vi "CreateWO-CreateFolderOnNetwork.vi"(8 "error in (no error)":errorcluster, 9 "Sales Order":string="1234", 10 "Work Order":string="1234", 11 "NI_report in":refnum<class "NI_report.lvclass">) -> (0 "error out":errorcluster, 1 "Work Order":string, 2 "Path for Saving the file":path, 3 "NI_report out":refnum<class "NI_report.lvclass">, 5 "Path for Outlook":path)   [LabVIEW 2013, in "ERP-CreateWorkOrder.lvclass"]
uses:
  ERP-CreateWorkOrder.lvclass
  <vilib>/Utility/NIReport.llb/NI_report.lvclass
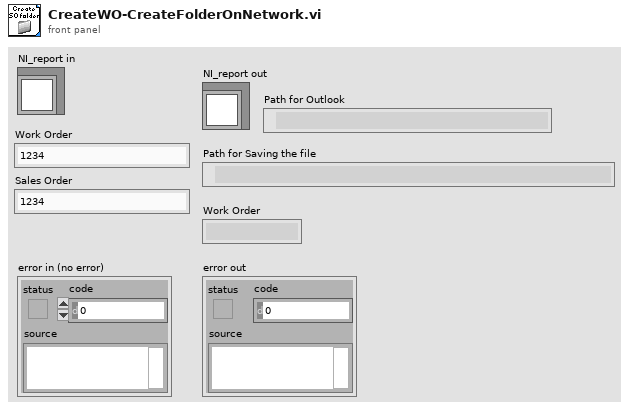
[diagram p1: front panel]
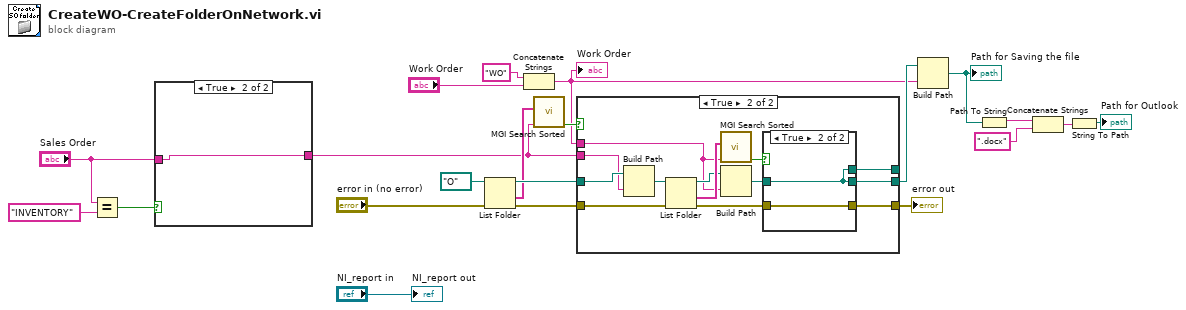
[diagram p0: block diagram]
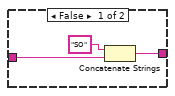
[diagram p2: hidden frame]
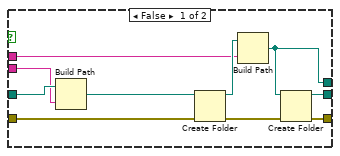
[diagram p3: hidden frame]
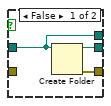
[diagram p4: hidden frame]
diagram:
  n1 = Equal?(x="Sales Order", y="INVENTORY") -> (x = y?=w6:bool)
  n2 = case shown="True" w6 {
    tunnel: "Sales Order" -> [w23 w25]
    tunnel: [w22 w25] -> w12
    frame False {
      n3 = Concatenate Strings("SO" ("string"), w23) -> (w22:string)
    }
    frame True {
    }
  }
  n4 = List Folder(path=path "O:/" ("base path"), error in="error in (no error)") -> (path out=w18:path, folder names=w14:string[], error out=w19:errorcluster)  [unwired: 2 in, 1 out]
  n5 = Concatenate Strings("WO" ("string"), "Work Order") -> (w9:string)
  "Work Order" <- w9
  n6 = call <userlib>:"MGI Search Sorted.vi"("Search String"=w12, "Sorted Strings"=w14) -> ("Found"=w13:bool)  [unwired: 6 in, 3 out]
  n7 = case shown="True" w13 {
    tunnel: w19 -> [w32 w44]
    tunnel: w18 -> [w34 w46]
    tunnel: [w27 w48] -> w17
    tunnel: [w28 w47] -> w16
    tunnel: w9 -> [w29 w38]
    tunnel: w12 -> [w33 w45]
    tunnel: [w26 w36] -> _
    frame False {
      n8 = Build Path(base path=w34, name or relative path=w33) -> (appended path=w35:path)
      n9 = Create Folder(path (use dialog)=w35, error in=w32) -> (created path=w30:path, error out=w31:errorcluster)  [unwired: 1 in, 1 out]
      n10 = Build Path(base path=w30, name or relative path=w29) -> (appended path=w26:path)
      n11 = Create Folder(path (use dialog)=w26, error in=w31) -> (created path=w28:path, error out=w27:errorcluster)  [unwired: 1 in, 1 out]
    }
    frame True {
      n12 = Build Path(base path=w46, name or relative path=w45) -> (appended path=w40:path)
      n13 = List Folder(path=w40, error in=w44) -> (path out=w39:path, folder names=w43:string[], error out=w41:errorcluster)  [unwired: 2 in, 1 out]
      n14 = call <userlib>:"MGI Search Sorted.vi"("Search String"=w38, "Sorted Strings"=w43) -> ("Found"=w42:bool)  [unwired: 6 in, 3 out]
      n15 = Build Path(base path=w39, name or relative path=w38) -> (appended path=w37:path)
      n16 = case shown="True" w42 {
        tunnel: [w51 w53] -> w48
        tunnel: [w50 w52] -> w47
        tunnel: w37 -> [w49 w52]
        tunnel: w41 -> [_ w53]
        tunnel: [w49 w52] -> w36
        frame False {
          n17 = Create Folder(path (use dialog)=w49) -> (created path=w50:path, error out=w51:errorcluster)  [unwired: 2 in, 1 out]
        }
        frame True {
        }
      }
    }
  }
  "error out" <- w17
  n18 = Build Path(base path=w16, name or relative path=w9) -> (appended path=w5:path)
  "Path for Saving the file" <- w5
  n19 = Path To String(path=w5) -> (string=w4:string)
  n20 = Concatenate Strings(w4, ".docx" ("string")) -> (w2:string)
  n21 = String To Path(string=w2) -> (path=→"Path for Outlook":path)
  "NI_report out" <- "NI_report in"
